vi "diameter of pipe.vi"() -> ()   [LabVIEW 2014]
uses:
  <vilib>/vision/NI_Vision_Development_Module.lvlib
panel:
  out "The diameter":dbl[](array[numeric])
  out "subarray":dbl[](array[numeric])
  out "Particle Measurements (Pixels) (Particle Analysis 1)":dbl[][](array[numeric]) format="%.2f"
  out "Image from IMAQ cast":T1(plugin-control)
  out "Image after colour palette":T1(plugin-control)
  out "Image from IMAQ extract tetragon":T1(plugin-control)
  out "Image":T1(plugin-control)
  out "Image from  Vision Acquisition 1":T1(plugin-control)
  out "Image from Vision Acquisition 2":T1(plugin-control)
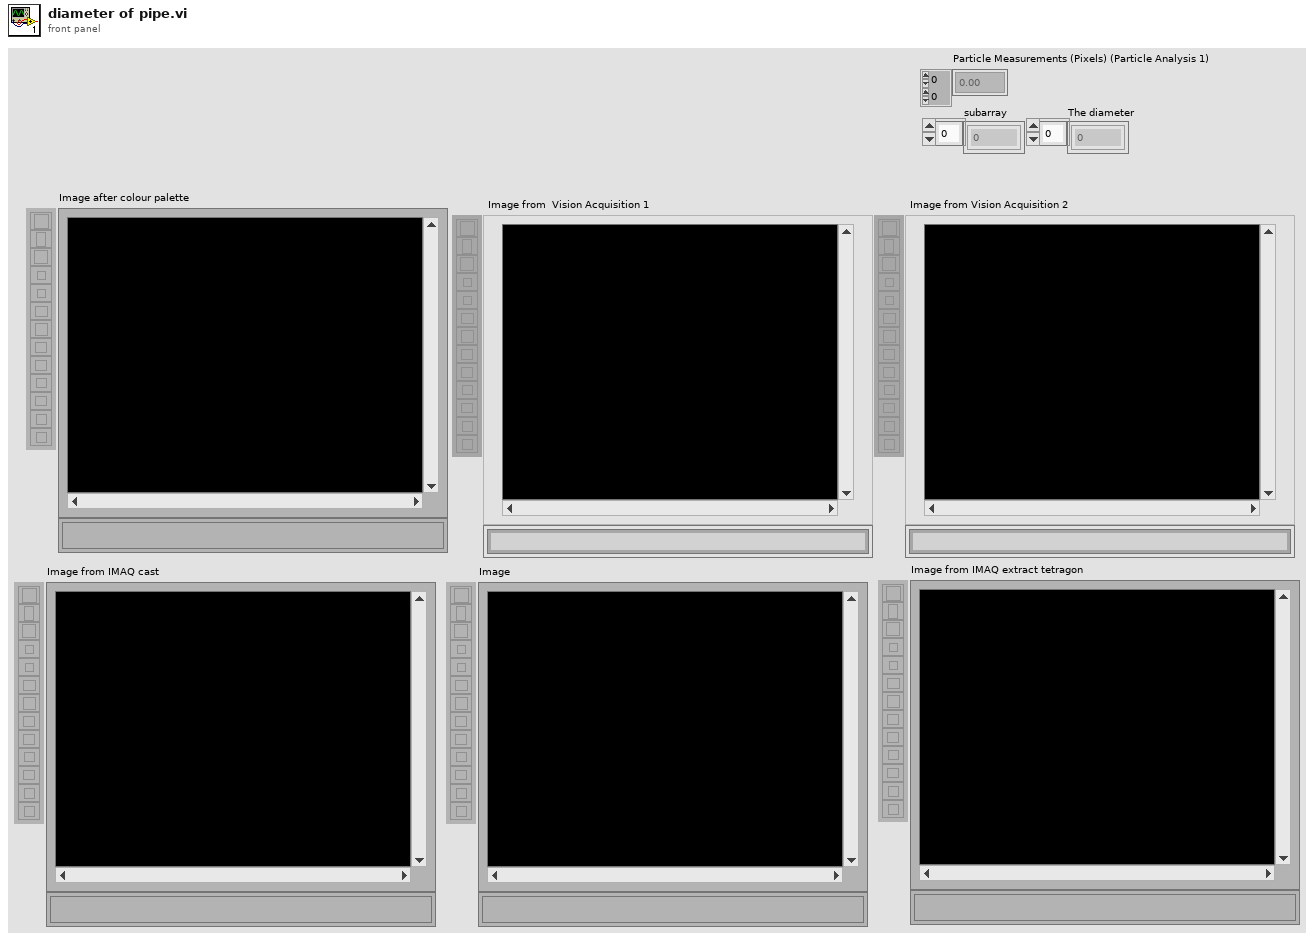
[diagram p1: front panel]
types:
  T1 = typedef "IMAQ Image.ctl" = refnum<image>
  T2 = typedef "Board Id" = u8
  T3 = typedef "ROI Descriptor" = cluster{"Global Rectangle":i32[], "Contours":cluster{"ID":enum32{"External", "Internal"}, "Type":u32, "Coordinates":i32[]}[]}
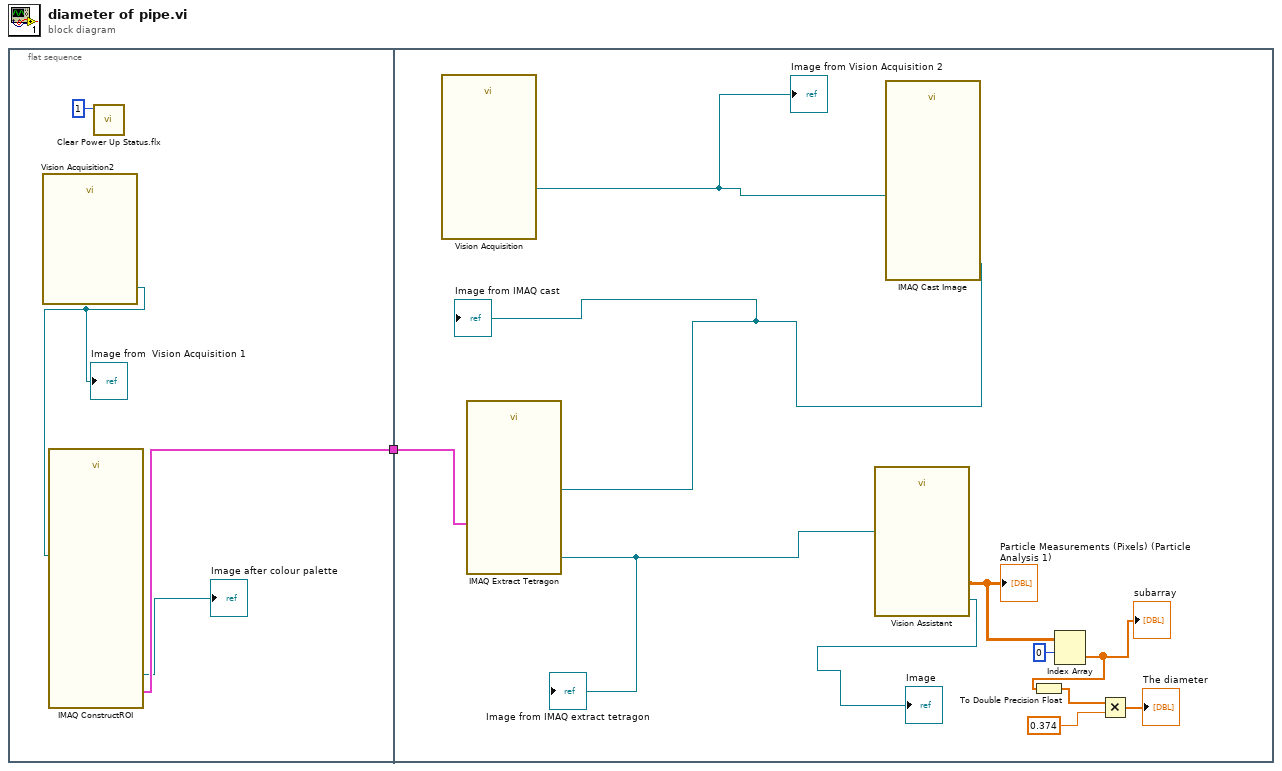
[diagram p0: block diagram]
diagram:
  n1 = flat-sequence {
    tunnel: [w5] -> w1
    tunnel: w1 -> [w16]
    frame #0 {
      n2 = call "Vision Acquisition2"() -> ("Image Out"=w3:T1)  [unwired: 25 in, 2 out]
      "Image from  Vision Acquisition 1" <- w3
      n3 = call "IMAQ ConstructROI"("Image"=w3) -> ("ROI Descriptor Out"=w5:T3, "Image Out (duplicate)"=→"Image after colour palette":T1)  [unwired: 7 in, 2 out]
      n4 = call <vilib>:"Clear Power Up Status.flx"("Board ID"=T2 1) -> ()  [unwired: 6 in, 2 out]
    }
    frame #1 {
      n5 = call "Vision Acquisition"() -> ("Image Out"=w14:T1)  [unwired: 25 in, 2 out]
      "Image from Vision Acquisition 2" <- w14
      n6 = call "IMAQ Cast Image"("Image Src"=w14) -> ("Image Dst Out"=w12:T1)  [unwired: 9 in, 1 out]
      "Image from IMAQ cast" <- w12
      n7 = call-poly "IMAQ Extract Tetragon"("ROI Descriptor"=w16, "Image Src"=w12) -> ("Image Dst Out"=w13:T1)  [unwired: 8 in, 1 out]
      "Image from IMAQ extract tetragon" <- w13
      n8 = call "Vision Assistant"("Image In"=w13) -> ("Image Out"=→"Image":T1, "Particle Measurements (Pixels) (Particle Analysis 1)"=w11:dbl[][])  [unwired: 23 in, 2 out]
      "Particle Measurements (Pixels) (Particle Analysis 1)" <- w11
      n9 = Index Array(array=w11, index (row)=0) -> (element=w9:dbl[])  [unwired: 1 in]
      "subarray" <- w9
      n10 = To Double Precision Float(number=w9) -> (double precision float=w8:dbl[])
      n11 = Multiply(x=w8, y=0.374) -> (x*y=→"The diameter":dbl[])
    }
  }
